vi "Length_3_R2.vi"() -> ()   [LabVIEW 2020]
uses:
  Support/Controls/Cmd_Mouse Popup.ctl
  Support/Controls/Clst_Initialize Input.ctl
  Support/Controls/Clst_Result inspec.ctl
  Support/Controls/Cmd_Var Data IO.ctl
  Variables/Global_Cal Info.vi
panel:
  out "최소범위":string
  in  "Measured_ADJ":string[][](table) caption="조정후"
  in  "구분":string(combo)
  in  "Measured 2":string[][](table) caption="1. 거칠기 측정 조건 & 잔류잡음 측정"
  in  "표시방식":string(combo)
  out "단위":string
  out "최대범위":string
  in  "Spec 변경":bool
  in  "Random":bool
  out "Resolution":string[][](table) caption="Spec"
  out "Spec":string[][](table)
  out "제목":string
  out "에러 출력":errorcluster
  out "Condition":string[][](table) caption="2. 직선성 시험"
  in  "최소눈금":string(combo)
  in  "Measured":string[][](table) caption="조정전"
  out "Load?":bool
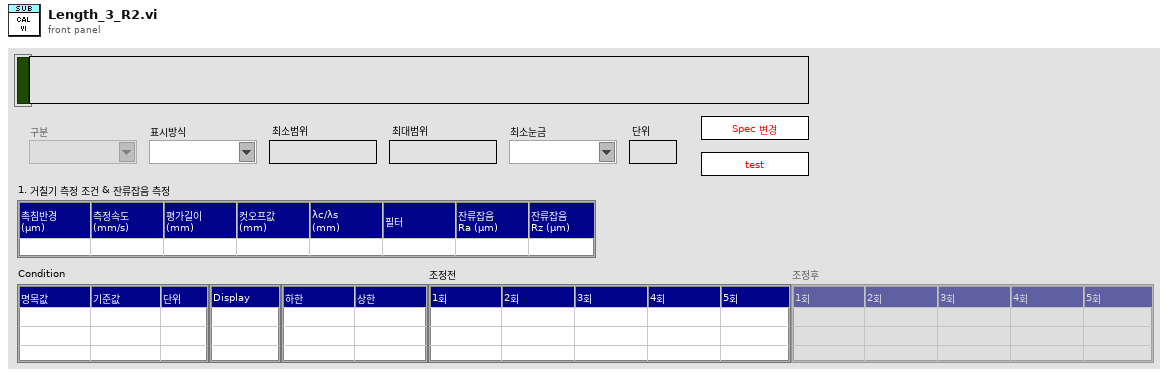
[diagram p1: front panel]
types:
  T1 = typedef "Cmd_Mouse Popup.ctl" = enum16{"활성화", "메뉴선택"}
  T2 = cluster{"Shift":bool, "Ctrl":bool, "Alt":bool, "Cmd":bool, "Opt":bool}
  T3 = typedef "Clst_Initialize Input.ctl" = cluster{"Initialize 1":cluster{"Condition":refnum<vi>[], "Spec":refnum<vi>[], "Measured":refnum<vi>[], "Resolution":refnum<vi>[], "Func_ext":string, "제목":refnum<vi>, "Measured_ADJ":refnum<vi>[]}, "Initialize 2":cluster{"문자열":refnum<vi>[], "콤보박스":refnum<vi>[], "링":refnum<vi>[], "열거형":refnum<vi>[], "테이블":refnum<vi>[], "여러열":refnum<vi>[], "디지털(DBL)":refnum<vi>[], "3D string":refnum<vi>[], "ctrl":refnum<vi>[], "boolean":refnum<vi>[]}}
  T4 = enum8{"Enabled", "Disabled", "Disabled and Grayed Out"}
  T5 = typedef "Clst_Result inspec.ctl" = cluster{"분해능":string, "문자열 1":string, "문자열 2":string, "숫자형 1":i32, "숫자형 2":i32, "숫자형 3":dbl, "문자배열 1D":string[], "문자배열 2D":string[][], "문자배열 3D":string[][][], "문자배열 4D":string[][][][], "불리언 1D":bool[]}
  T6 = typedef "Cmd_Var Data IO.ctl" = enum16{"Condition", "Condition Default", "Condition_Temp", "Resolution", "Resolution Default", "Resolution Old", "Spec", "Spec Default", "Spec Old", "Spec Temp", "Result", "Result2", "Result3", "Result_Temp", "Result_ADJ", "Result_ADJ2", "STD1", "STD2", "STD3", "STD4", "STD5", "STD Temp", "CMC", "CMC Default"}
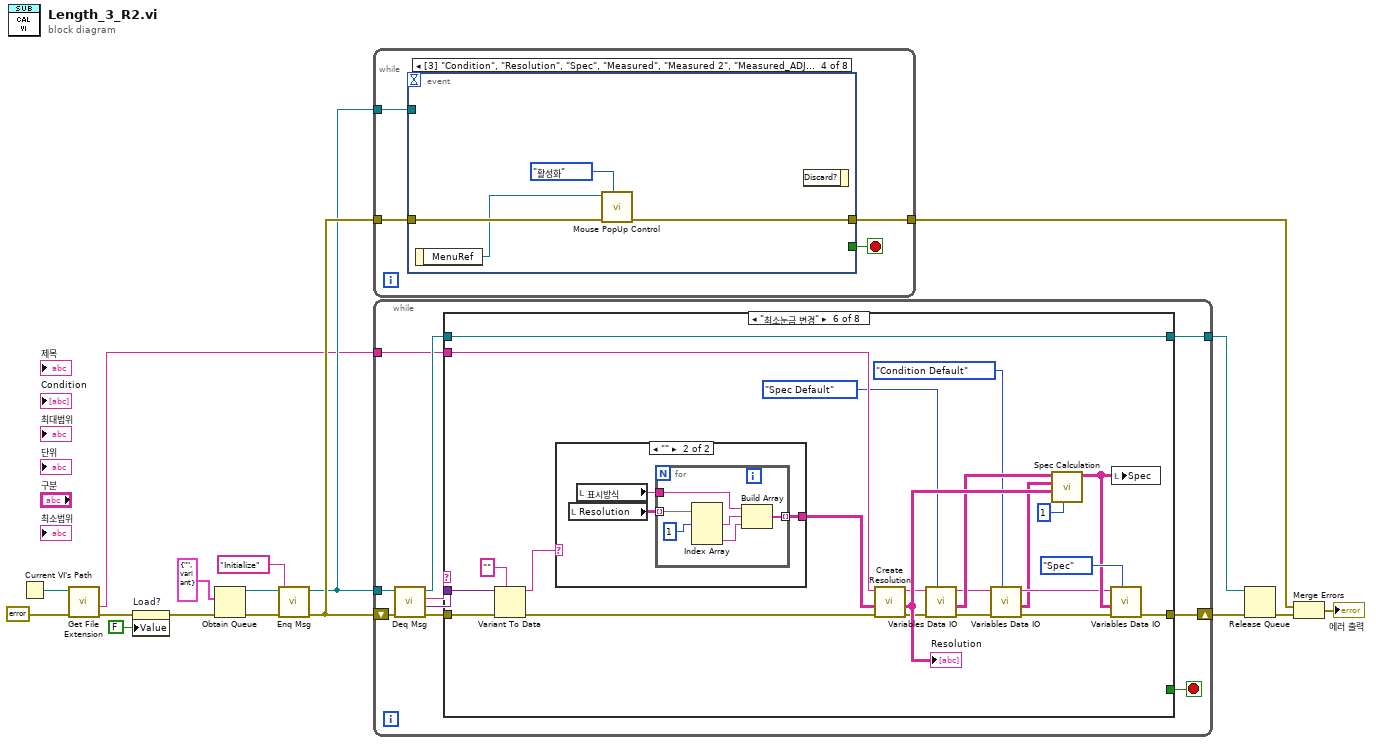
[diagram p0: block diagram]
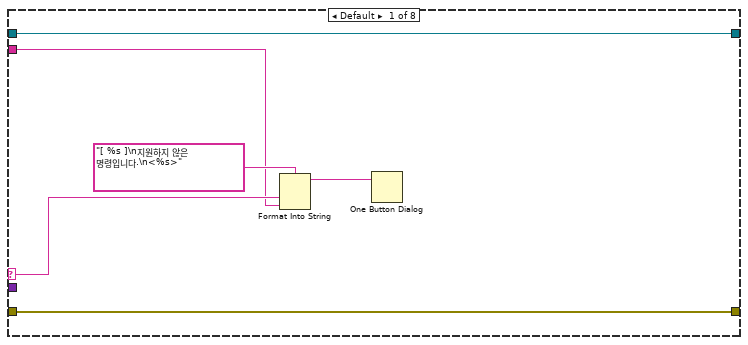
[diagram p2: hidden frame]
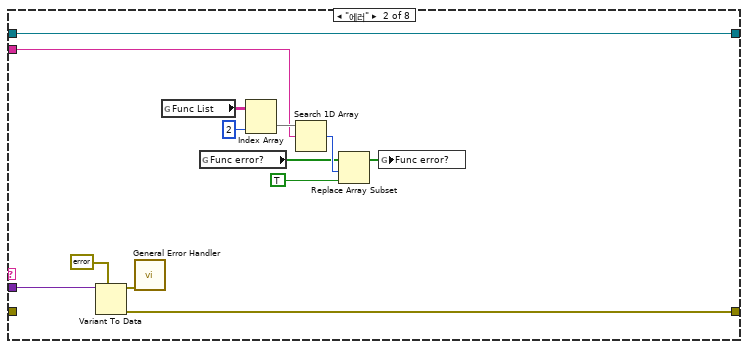
[diagram p3: hidden frame]
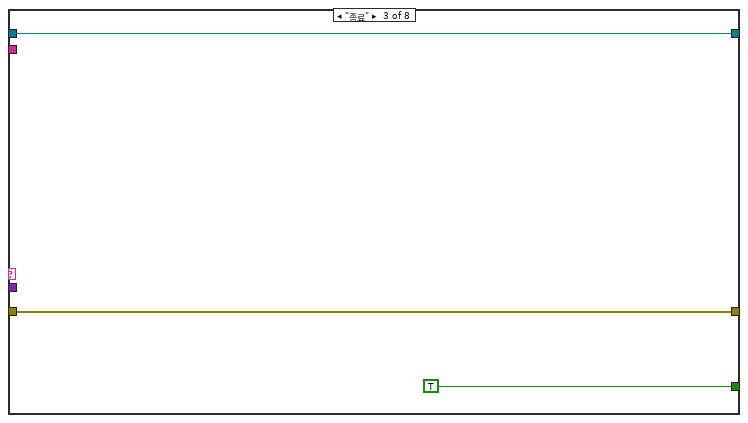
[diagram p4: hidden frame]
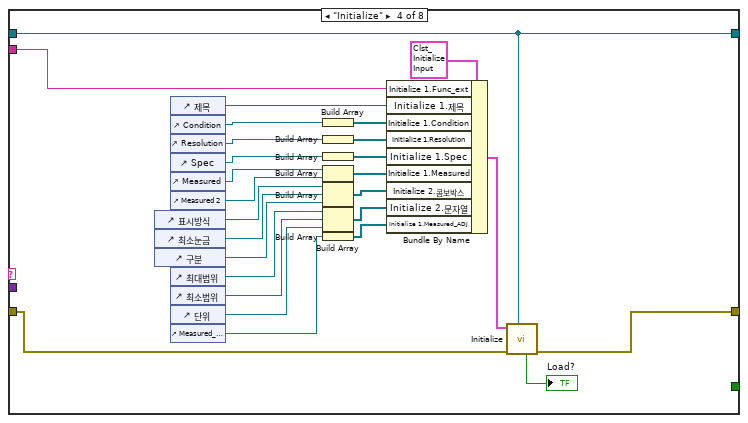
[diagram p5: hidden frame]
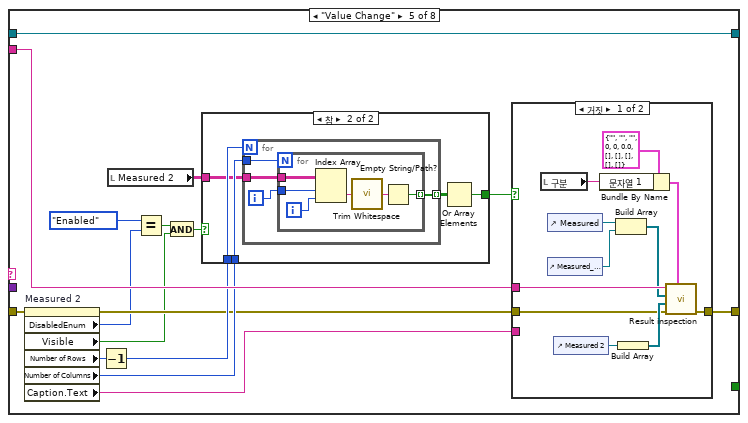
[diagram p6: hidden frame]
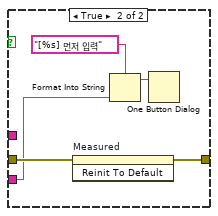
[diagram p8: hidden frame]
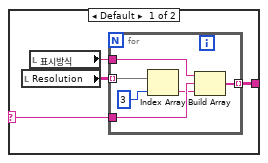
[diagram p9: hidden frame]
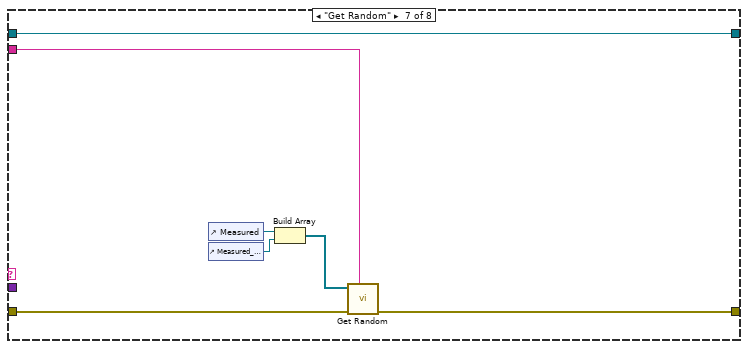
[diagram p10: hidden frame]
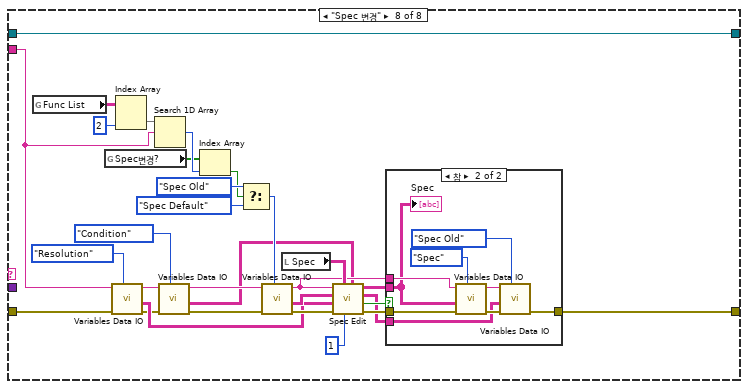
[diagram p11: hidden frame]
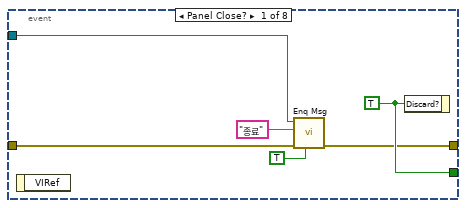
[diagram p13: hidden frame]
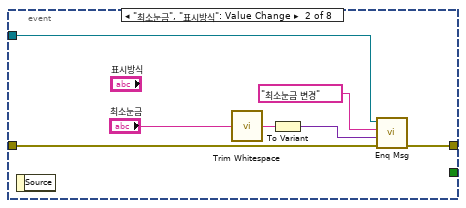
[diagram p14: hidden frame]
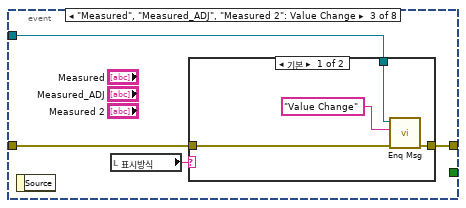
[diagram p15: hidden frame]
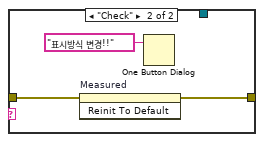
[diagram p16: hidden frame]
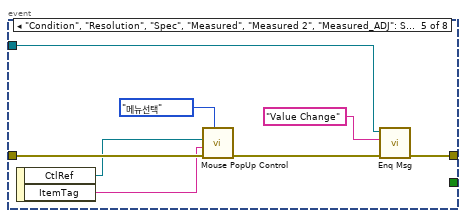
[diagram p17: hidden frame]
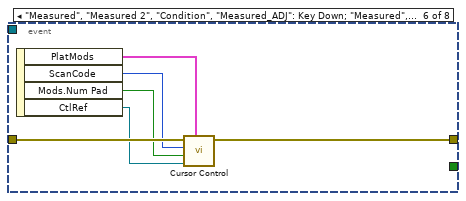
[diagram p18: hidden frame]
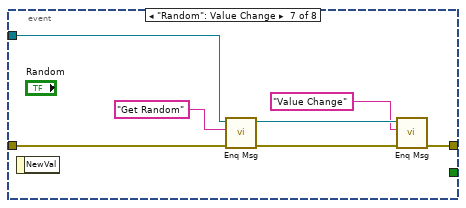
[diagram p19: hidden frame]
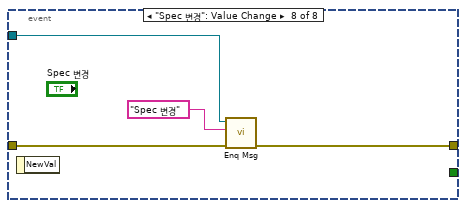
[diagram p20: hidden frame]
diagram:
  n1 = Current VI's Path() -> (path=w5:path)
  n2 = call <vilib>:"Get File Extension.vi"("error in (no error)"=errorcluster {"status"=FALSE, "code"=0, "source"=""} ("에러 상수"), "file"=w5) -> ("error out"=w3:errorcluster, "filename without extension"=w4:string)  [unwired: 5 in, 3 out]
  n3 = property on="Load?" class="Bool (엄격한)"(error in=w3, "Value"=FALSE ("Load?")) -> (error out=w2:errorcluster)  [unwired: 1 in, 1 out]
  n4 = Obtain Queue(element data type=cluster{"메세지":string, "값":variant} {"메세지"="", "값"=variant} ("Message Cluster"), error in (no error)=w2) -> (queue out=w14:refnum<queue>, error out=w16:errorcluster)  [unwired: 3 in, 1 out]
  n5 = call "Enq Msg.vi"("에러 입력(에러 없음)"=w16, "메세지"="Initialize", "큐 입력"=w14) -> ("에러 출력"=w15:errorcluster, "큐 출력"=w12:refnum<queue>)  [unwired: 7 in]
  n6 = while {
    tunnel: w15 -> [w19]
    tunnel: w12 -> [w20]
    tunnel: [w18] -> w9
    stop <- w21 stop-if-true
    n7 = event shown="[3] \"Condition\", \"Resolution\", \"Spec\", \"Measured\", \"Measured 2\", \"Measured_ADJ\": 바로 가기 메뉴 활성화?" {
      selector: _ -> [_ _ _ _ _ _ _ _]
      dyn-events: _ -> [_ _ _ _ _ _ _ _]
      timeout: _ -> [_ _ _ _ _ _ _ _]
      tunnel: [w27 _ _ _ _ _ _ _] -> w21
      tunnel: w20 -> [w25 w33 w38 _ w50 _ w68 w72]
      tunnel: w19 -> [w26 w34 w36 w49 w57 w63 w69 w73]
      tunnel: [w23 w32 w37 w48 w51 w62 w64 w71] -> w18
      event Panel Close? {
        w27 = TRUE ("버림?")
        n8 = event-data() -> ()  [unwired: 1 in, 1 out]
        n9 = call "Enq Msg.vi"("우선순위 메시지?"=TRUE, "에러 입력(에러 없음)"=w26, "메세지"="종료", "큐 입력"=w25) -> ("에러 출력"=w23:errorcluster)  [unwired: 6 in, 1 out]
        n10 = event-data("Discard?"=w27) -> ()  [unwired: 1 in, 1 out]
      }
      event "최소눈금", "표시방식": Value Change {
        n11 = event-data() -> ()  [unwired: 1 in, 1 out]
        n12 = call <vilib>:"Trim Whitespace.vi"("string"="최소눈금") -> ("trimmed string"=w30:string)  [unwired: 1 in]
        n13 = To Variant(anything=w30) -> (Variant=w28:variant)
        n14 = call "Enq Msg.vi"("에러 입력(에러 없음)"=w34, "값"=w28, "메세지"="최소눈금 변경", "큐 입력"=w33) -> ("에러 출력"=w32:errorcluster)  [unwired: 6 in, 1 out]
      }
      event "Measured", "Measured_ADJ", "Measured 2": Value Change {
        n15 = event-data() -> ()  [unwired: 1 in, 1 out]
        n16 = local read "표시방식"() -> (w35:string)
        n17 = case shown="기본" w35 {
          tunnel: w38 -> [w42 _]
          tunnel: [w41 w43] -> w37
          tunnel: w36 -> [w40 w44]
          frame Default {
            n18 = call "Enq Msg.vi"("에러 입력(에러 없음)"=w40, "메세지"="Value Change", "큐 입력"=w42) -> ("에러 출력"=w41:errorcluster)  [unwired: 7 in, 1 out]
          }
          frame "Check" {
            n19 = invoke on="Measured" class="Tbl (엄격한)" method="Reinit To Default"(error in=w44) -> (error out=w43:errorcluster)  [unwired: 2 in, 2 out]
            n20 = One Button Dialog(message="표시방식 변경!!" ("메시지")) -> ()  [unwired: 1 in, 1 out]
          }
        }
      }
      event "Condition", "Resolution", "Spec", "Measured", "Measured 2", "Measured_ADJ": Shortcut Menu Activation? {
        n21 = event-data() -> ("MenuRef"=w47:refnum<k9>)  [unwired: 1 in]
        n22 = call "Mouse PopUp Control.vi"("type"=Cmd_Mouse_Popup."활성화", "error in"=w49, "메뉴 참조"=w47) -> ("error out"=w48:errorcluster)  [unwired: 8 in]
        n23 = event-data() -> ()  [unwired: 2 in, 1 out]
      }
      event "Condition", "Resolution", "Spec", "Measured", "Measured 2", "Measured_ADJ": Shortcut Menu Selection (User) {
        n24 = event-data() -> ("CtlRef"=w55:refnum<vi>, "ItemTag"=w54:string)  [unwired: 1 in]
        n25 = call "Mouse PopUp Control.vi"("type"=Cmd_Mouse_Popup."메뉴선택", "error in"=w57, "아이템 태그"=w54, "Tbl 참조 번호"=w55) -> ("error out"=w52:errorcluster)  [unwired: 7 in]
        n26 = call "Enq Msg.vi"("에러 입력(에러 없음)"=w52, "메세지"="Value Change", "큐 입력"=w50) -> ("에러 출력"=w51:errorcluster)  [unwired: 7 in, 1 out]
      }
      event "Measured", "Measured 2", "Condition", "Measured_ADJ": Key Down; "Measured", "Measured 2", "Condition", "Measured_ADJ": Key Repeat {
        n27 = event-data() -> ("PlatMods"=w58:T2, "ScanCode"=w61:i16, "Mods.Num Pad"=w60:bool, "CtlRef"=w59:refnum<vi>)  [unwired: 1 in]
        n28 = call "Cursor Control.vi"("플랫폼 조합키"=w58, "참조"=w59, "Num Pad"=w60, "ScanCode"=w61, "error in"=w63) -> ("error out"=w62:errorcluster)  [unwired: 5 in, 1 out]
      }
      event "Random": Value Change {
        n29 = event-data() -> ()  [unwired: 1 in, 1 out]
        n30 = call "Enq Msg.vi"("에러 입력(에러 없음)"=w69, "메세지"="Get Random", "큐 입력"=w68) -> ("에러 출력"=w67:errorcluster, "큐 출력"=w66:refnum<queue>)  [unwired: 7 in]
        n31 = call "Enq Msg.vi"("에러 입력(에러 없음)"=w67, "메세지"="Value Change", "큐 입력"=w66) -> ("에러 출력"=w64:errorcluster)  [unwired: 7 in, 1 out]
      }
      event "Spec 변경": Value Change {
        n32 = event-data() -> ()  [unwired: 1 in, 1 out]
        n33 = call "Enq Msg.vi"("에러 입력(에러 없음)"=w73, "메세지"="Spec 변경", "큐 입력"=w72) -> ("에러 출력"=w71:errorcluster)  [unwired: 7 in, 1 out]
      }
    }
  }
  n34 = while {
    shift-right: [w84] -> w11
    shift-left: w15 -> [w83]
    tunnel: w12 -> [w81]
    tunnel: [w76] -> w10
    tunnel: w4 -> [w75]
    stop <- w77 stop-if-true
    n35 = call "Deq Msg.vi"("에러 입력(에러 없음)"=w83, "큐 입력"=w81) -> ("에러 출력"=w82:errorcluster, "값"=w78:variant, "메세지"=w80:string, "큐 출력"=w79:refnum<queue>)  [unwired: 6 in]
    n36 = case shown="\"최소눈금 변경\"" w80 {
      selector: w80 -> [w86 _ _ _ _ _ _ _]
      tunnel: w82 -> [w90 _ w106 w133 w146 w202 w225 w252]
      tunnel: [w90 w100 w106 w123 w148 w195 w226 w255] -> w84
      tunnel: w79 -> [w89 w99 w104 w117 w149 w203 w229 w259]
      tunnel: w78 -> [_ w101 _ _ _ w201 _ _]
      tunnel: [_ _ TRUE ("버림?") _ _ _ _ _] -> w77
      tunnel: [w89 w99 w104 w117 w149 w203 w229 w259] -> w76
      tunnel: w75 -> [w85 w91 _ w118 w147 w199 w224 w237]
      frame Default {
        n37 = Format Into String(format string="[ %s ]\n지원하지 않은 명령입니다.\n<%s>" ("메시지"), w86, w85) -> (resulting string=w87:string)  [unwired: 2 in, 1 out]
        n38 = One Button Dialog(message=w87) -> ()  [unwired: 1 in, 1 out]
      }
      frame "에러" {
        n39 = Variant To Data(type=errorcluster {"status"=FALSE, "code"=0, "source"=""} ("에러 출력"), Variant=w101) -> (data=w103:errorcluster, error out=w100:errorcluster)  [unwired: 1 in]
        n40 = call <vilib>:"General Error Handler.vi"("error in (no error)"=w103) -> ()  [unwired: 10 in, 5 out]
        n41 = global read "Global_Cal Info.vi" "Func List"() -> (w93:string[][])
        n42 = global read "Global_Cal Info.vi" "Func error?"() -> (w96:bool[])
        n43 = Index Array(array=w93, index (col)=2 ("비활성화된 인덱스 (열)")) -> (element=w94:string[])  [unwired: 1 in]
        n44 = Search 1D Array(1D array=w94, element=w91) -> (index of element=w97:i32)  [unwired: 1 in]
        n45 = Replace Array Subset(array=w96, new element=TRUE ("새 원소/부분배열"), index=w97) -> (w98:bool[])
        n46 = global write "Global_Cal Info.vi" "Func error?"(w98) -> ()
      }
      frame "종료" {
      }
      frame "Initialize" {
        n47 = control-ref of="표시방식"() -> (w116:refnum<vi>)
        n48 = control-ref of="최소눈금"() -> (w126:refnum<vi>)
        n49 = control-ref of="구분"() -> (w112:refnum<vi>)
        n50 = control-ref of="제목"() -> (w124:refnum<vi>)
        n51 = control-ref of="Condition"() -> (w130:refnum<vi>)
        n52 = control-ref of="Resolution"() -> (w119:refnum<vi>)
        n53 = control-ref of="Spec"() -> (w122:refnum<vi>)
        n54 = control-ref of="Measured"() -> (w127:refnum<vi>)
        n55 = control-ref of="Measured 2"() -> (w107:refnum<vi>)
        n56 = control-ref of="최대범위"() -> (w113:refnum<vi>)
        n57 = control-ref of="최소범위"() -> (w108:refnum<vi>)
        n58 = control-ref of="단위"() -> (w115:refnum<vi>)
        n59 = control-ref of="Measured_ADJ"() -> (w111:refnum<vi>)
        n60 = Build Array(w130) -> (w129:refnum<vi>[])
        n61 = Build Array(w119) -> (w120:refnum<vi>[])
        n62 = Build Array(w122) -> (w121:refnum<vi>[])
        n63 = Build Array(w127, w107) -> (w128:refnum<vi>[])
        n64 = Build Array(w116, w126, w112) -> (w125:refnum<vi>[])
        n65 = Build Array(w113, w108, w115) -> (w114:refnum<vi>[])
        n66 = Build Array(w111) -> (w110:refnum<vi>[])
        n67 = Bundle By Name(cluster=T3 {"Initialize 1"={"Condition"=[], "Spec"=[], "Measured"=[], "Resolution"=[], "Func_ext"="", "제목"=refnum, "Measured_ADJ"=[]}, "Initialize 2"={"문자열"=[], "콤보박스"=[], "링"=[], "열거형"=[], "테이블"=[], "여러열"=[], "디지털(DBL)"=[], "3D string"=[], "ctrl"=[], "boolean"=[]}} ("입력 클러스터"), "Initialize 1.Func_ext"=w118, "Initialize 1.제목"=w124, "Initialize 1.Condition"=w129, "Initialize 1.Resolution"=w120, "Initialize 1.Spec"=w121, "Initialize 1.Measured"=w128, "Initialize 2.콤보박스"=w125, "Initialize 2.문자열"=w114, "Initialize 1.Measured_ADJ"=w110) -> (w131:T3)
        n68 = call "Initialize.vi"("큐 입력"=w117, "error in"=w133, "입력 클러스터"=w131) -> ("error out"=w123:errorcluster, "Load?"=→"Load?":bool)  [unwired: 5 in, 2 out]
      }
      frame "Value Change" {
        n69 = property on="Measured 2" class="Tbl (엄격한)"(error in=w146) -> (error out=w142:errorcluster, "DisabledEnum"=w137:T4, "Visible"=w139:bool, "Number of Rows"=w140:u32, "Number of Columns"=w145:u32, "Caption.Text"=w141:string)  [unwired: 1 in, 1 out]
        n70 = Decrement(x=w140) -> (x-1=w144:u32)
        n71 = local read "Measured 2"() -> (w134:string[][])
        n72 = Equal?(x=T4."Enabled" ("비활성화"), y=w137) -> (x = y?=w135:bool)
        n73 = And(x=w135, y=w139) -> (x .and. y?=w136:bool)
        n74 = case shown="참" w136 {
          tunnel: w145 -> [_ w154]
          tunnel: w144 -> [_ w153]
          tunnel: [_ w151] -> w143
          tunnel: w134 -> [_ w150]
          frame False {
          }
          frame True {
            n75 = for {
              N: w153 -> [_]
              tunnel: w150 -> [w157]
              tunnel: w154 -> [w158]
              tunnel: [w155] -> w152 mode=indexing
              i -> [w156]
              n76 = for {
                N: w158 -> [_]
                tunnel: w157 -> [w164]
                tunnel: w156 -> [w163]
                tunnel: [w159] -> w155 mode=indexing
                i -> [w162]
                n77 = Index Array(array=w164, index (row)=w163, index (col)=w162) -> (element=w161:string)
                n78 = call <vilib>:"Trim Whitespace.vi"("string"=w161) -> ("trimmed string"=w160:string)  [unwired: 1 in]
                n79 = Empty String/Path?(string/path=w160) -> (empty?=w159:bool)
              }
            }
            n80 = Or Array Elements(Boolean array=w152) -> (logical OR=w151:bool)
          }
        }
        n81 = case shown="거짓" w143 {
          tunnel: [w175 w179] -> w148
          tunnel: w147 -> [w174 _]
          tunnel: w142 -> [w167 w180]
          tunnel: w141 -> [_ w176]
          frame False {
            n82 = local read "구분"() -> (w165:string)
            n83 = control-ref of="Measured"() -> (w173:refnum<vi>)
            n84 = control-ref of="Measured_ADJ"() -> (w166:refnum<vi>)
            n85 = control-ref of="Measured 2"() -> (w169:refnum<vi>)
            n86 = Bundle By Name(cluster=T5 {"분해능"="", "문자열 1"="", "문자열 2"="", "숫자형 1"=0, "숫자형 2"=0, "숫자형 3"=0.0, "문자배열 1D"=[], "문자배열 2D"=[], "문자배열 3D"=[], "문자배열 4D"=[], "불리언 1D"=[]} ("입력 클러스터"), "문자열 1"=w165) -> (w170:T5)
            n87 = Build Array(w173, w166) -> (w172:refnum<vi>[])
            n88 = Build Array(w169) -> (w168:refnum<vi>[])
            n89 = call "Result inspection.vi"("입력 클러스터"=w170, "error in"=w167, "Ref. Data (excluded)"=w168, "Ref. Data (Inspection)"=w172, "Func ext"=w174) -> ("error out"=w175:errorcluster)  [unwired: 3 in, 3 out]
          }
          frame True {
            n90 = invoke on="Measured" class="Tbl (엄격한)" method="Reinit To Default"(error in=w180) -> (error out=w179:errorcluster)  [unwired: 2 in, 2 out]
            n91 = Format Into String(format string="[%s] 먼저 입력" ("포맷 문자열"), w176) -> (resulting string=w178:string)  [unwired: 2 in, 1 out]
            n92 = One Button Dialog(message=w178) -> ()  [unwired: 1 in, 1 out]
          }
        }
      }
      frame "최소눈금 변경" {
        n93 = Variant To Data(error in=w202, type="", Variant=w201) -> (data=w188:string, error out=w190:errorcluster)
        n94 = case shown="\"\"" w188 {
          selector: w188 -> [w204 _]
          tunnel: [w207 w216] -> w189
          frame Default {
            n95 = local read "Resolution"() -> (w206:string[][])
            n96 = local read "표시방식"() -> (w205:string)
            n97 = for {
              tunnel: w206 -> [w213] mode=indexing
              tunnel: w204 -> [w212]
              tunnel: [w210] -> w207 mode=indexing
              tunnel: w205 -> [w209]
              n98 = Index Array(array=w213, index=3 ("인덱스")) -> (element=w211:string)
              n99 = Build Array(w209, w212, w211) -> (w210:string[])
            }
          }
          frame "" {
            n100 = local read "Resolution"() -> (w215:string[][])
            n101 = local read "표시방식"() -> (w214:string)
            n102 = for {
              tunnel: w215 -> [w222] mode=indexing
              tunnel: [w221] -> w216 mode=indexing
              tunnel: w214 -> [w220]
              n103 = Index Array(array=w222, index #1=1 ("인덱스")) -> (element #1=w218:string, element #3=w217:string)  [unwired: 2 in, 1 out]
              n104 = Build Array(w220, w218, w217) -> (w221:string[])
            }
          }
        }
        n105 = call "Create Resolution.vi"("에러 입력(에러 없음)"=w190, "Resolution"=w189, "Func_ext"=w199) -> ("에러 출력"=w193:errorcluster, "Resolution Out"=w196:string[][], "Func_ext 출력"=w192:string)  [unwired: 6 in]
        "Resolution" <- w196
        n106 = call "Variables Data IO.vi"("Select"=Cmd_Var_Data_IO."Spec Default", "error in"=w193, "Func_ext"=w192) -> ("error out"=w185:errorcluster, "Data Out"=w191:string[][], "Func_ext Out"=w184:string)  [unwired: 6 in]
        n107 = call "Variables Data IO.vi"("Select"=Cmd_Var_Data_IO."Condition Default", "error in"=w185, "Func_ext"=w184) -> ("error out"=w182:errorcluster, "Data Out"=w181:string[][], "Func_ext Out"=w183:string)  [unwired: 6 in]
        n108 = call "Spec Calculation.vi"("기준값 열번호"=1 ("열번호(기준값)"), "Resolution"=w196, "Condition in"=w181, "Spec Default"=w191) -> ("Spec out"=w187:string[][])  [unwired: 6 in, 1 out]
        n109 = call "Variables Data IO.vi"("Select"=Cmd_Var_Data_IO."Spec", "error in"=w182, "Data In"=w187, "Func_ext"=w183) -> ("error out"=w195:errorcluster)  [unwired: 5 in, 2 out]
        n110 = local write "Spec"(w187) -> ()
      }
      frame "Get Random" {
        n111 = control-ref of="Measured"() -> (w228:refnum<vi>)
        n112 = control-ref of="Measured_ADJ"() -> (w223:refnum<vi>)
        n113 = Build Array(w228, w223) -> (w227:refnum<vi>[])
        n114 = call "Get Random.vi"("Func_Ext"=w224, "에러 입력"=w225, "Meas"=w227) -> ("에러 출력"=w226:errorcluster)  [unwired: 7 in, 1 out]
      }
      frame "Spec 변경" {
        n115 = global read "Global_Cal Info.vi" "Func List"() -> (w242:string[][])
        n116 = global read "Global_Cal Info.vi" "Spec변경?"() -> (w238:bool[])
        n117 = call "Variables Data IO.vi"("Select"=Cmd_Var_Data_IO."Resolution", "error in"=w252, "Func_ext"=w237) -> ("error out"=w235:errorcluster, "Data Out"=w246:string[][], "Func_ext Out"=w233:string)  [unwired: 6 in]
        n118 = Index Array(array=w242, index (col)=2 ("비활성화된 인덱스 (열)")) -> (element=w240:string[])  [unwired: 1 in]
        n119 = Search 1D Array(1D array=w240, element=w237) -> (index of element=w239:i32)  [unwired: 1 in]
        n120 = call "Variables Data IO.vi"("Select"=Cmd_Var_Data_IO."Condition", "error in"=w235, "Func_ext"=w233) -> ("error out"=w234:errorcluster, "Data Out"=w230:string[][], "Func_ext Out"=w232:string)  [unwired: 6 in]
        n121 = Index Array(array=w238, index=w239) -> (element=w243:bool)
        n122 = Select(t=Cmd_Var_Data_IO."Spec Old" ("Select"), s=w243, f=Cmd_Var_Data_IO."Spec Default" ("Select")) -> (s? t:f=w236:T6)
        n123 = call "Variables Data IO.vi"("Select"=w236, "error in"=w234, "Func_ext"=w232) -> ("error out"=w254:errorcluster, "Data Out"=w247:string[][], "Func_ext Out"=w248:string)  [unwired: 6 in]
        n124 = local read "Spec"() -> (w249:string[][])
        n125 = call "Spec Edit.vi"("Condition"=w230, "열번호(기준값)"=1, "Spec Value"=w249, "에러 입력(에러 없음)"=w254, "Resolution"=w246, "Spec Default"=w247, "Func_ext"=w248) -> ("에러 출력"=w256:errorcluster, "변경?"=w257:bool, "Spec Default out"=w251:string[][], "Spec 출력"=w258:string[][])  [unwired: 1 in]
        n126 = case shown="참" w257 {
          tunnel: w258 -> [_ w266]
          tunnel: w256 -> [w260 w269]
          tunnel: [w260 w264] -> w255
          tunnel: w248 -> [_ w267]
          tunnel: w251 -> [_ w262]
          frame False {
          }
          frame True {
            n127 = call "Variables Data IO.vi"("Select"=Cmd_Var_Data_IO."Spec", "error in"=w269, "Data In"=w266, "Func_ext"=w267) -> ("error out"=w265:errorcluster, "Func_ext Out"=w263:string)  [unwired: 5 in, 1 out]
            n128 = call "Variables Data IO.vi"("Select"=Cmd_Var_Data_IO."Spec Old", "error in"=w265, "Data In"=w262, "Func_ext"=w263) -> ("error out"=w264:errorcluster)  [unwired: 5 in, 2 out]
            "Spec" <- w266
          }
        }
      }
    }
  }
  n129 = Release Queue(queue=w10, error in (no error)=w11) -> (error out=w8:errorcluster)  [unwired: 1 in, 2 out]
  n130 = Merge Errors(w9, w8) -> (→"에러 출력":errorcluster)
